vi "Start.vi"(8 "error in (no error)":errorcluster, 10 "Message in":refnum<class "StartMessage.lvclass">, 11 "Galvo in":refnum<class "ImagingModeSPIM.lvclass">) -> (0 "error out":errorcluster, 3 "Galvo out":refnum<class "ImagingModeSPIM.lvclass">)   [LabVIEW 2012, in "ImagingModeSPIM.lvclass"]
doc: "This member function is called when the statemachine in the run.vi receives an 'start' command. It relays the message to all observers of the component.\n\nOverride this member function in your derived class if you need additional start functionality (but don't forget to call the parent method)."
uses:
  ImagingModeSPIM.lvclass
  <vilib>/Distrio/Murmex/StartMessage/StartMessage.lvclass
  <vilib>/Distrio/Murmex/Murmex/Murmex.lvclass
  <vilib>/Distrio/Murmex/StartMessage/run mode enum.ctl
  <vilib>/Distrio/Murmex/ProceedMessage/ProceedMessage.lvclass
  ImagingModeSPIM.lvclass/ImagingModeSPIM.ctl
  <vilib>/Distrio/Murmex/StartMessage/Get run mode.vi
panel:
  # "This member function is called when the statemachine in the run.vi receives an 'start' command. It relays the message to all observers of the component.\n\nOverride this member function in your derived class if you need additional start functionality (but don't forget to call the parent method)."
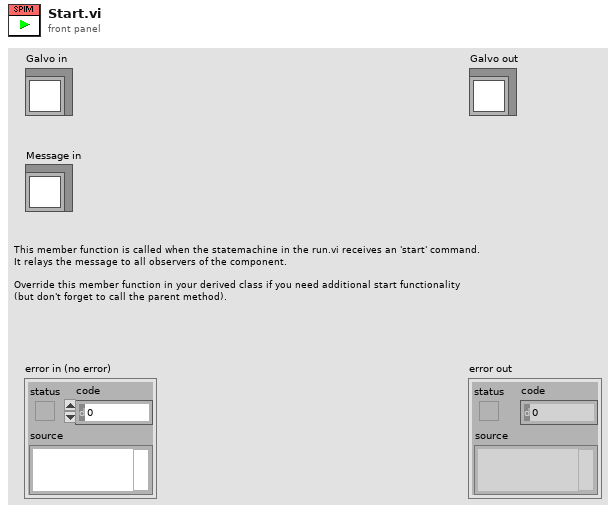
[diagram p1: front panel]
types:
  T1 = typedef "Murmex.lvlib/StartMessage.lvclass/run mode enum.ctl" = enum16{"infinite", "finite"}
  T2 = enum8{"Enabled", "Disabled", "Disabled and Grayed Out"}
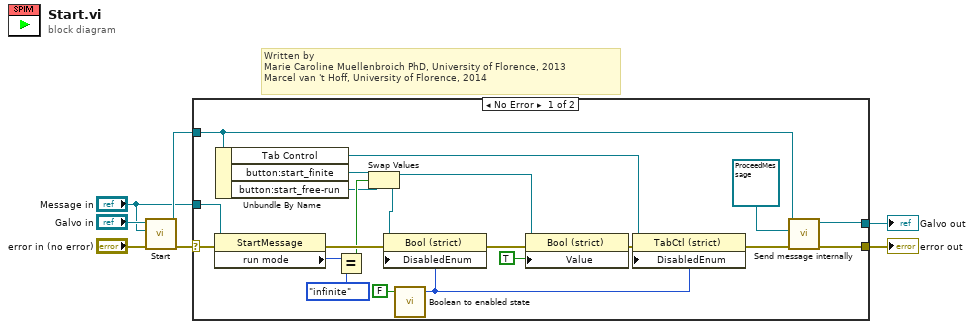
[diagram p0: block diagram]
diagram:
  # "Written by \nMarie Caroline Muellenbroich PhD, University of Florence, 2013 \nMarcel van 't Hoff, University of Florence, 2014"
  n1 = call-parent "Start.vi"("error in (no error)"="error in (no error)", "Message in"="Message in", "Murmex in"="Galvo in") -> ("error out"=w4:errorcluster, "Murmex out"=w5:refnum<class "ImagingModeSPIM.lvclass">)  [unwired: 7 in]
  n2 = case shown="No Error" w4 {
    selector: w4 -> [w25 w30]
    tunnel: w5 -> [w24 w29]
    tunnel: [w28 w30] -> w3
    tunnel: [w27 w29] -> w2
    tunnel: "Message in" -> [w26 _]
    frame No Error {
      n3 = property class="StartMessage"(reference=w26, error in=w25) -> (error out=w20:errorcluster, "run mode"=w23:T1)  [unwired: 1 out]
      n4 = Unbundle By Name(w24) -> ("Tab Control"=w19:refnum<vi>, "button:start_finite"=w15:refnum<vi>, "button:start_free-run"=w14:refnum<vi>)
      n5 = Equal?(x=w23, y=run_mode_enum."infinite" ("run mode")) -> (x = y?=w16:bool)
      n6 = Swap Values(12:w15, 13:w16, 14:w14) -> (1:w10:refnum<vi>, 3:w9:refnum<vi>)
      n7 = call <vilib>:"Boolean to enabled state.vi"("boolean in"=FALSE) -> ("enabled status out"=w18:T2)  [unwired: 4 in]
      n8 = property class="Bool (strict)"(reference=w9, error in=w20, "DisabledEnum"=w18) -> (error out=w12:errorcluster)  [unwired: 1 out]
      n9 = property class="Bool (strict)"(reference=w10, error in=w12, "Value"=TRUE) -> (error out=w11:errorcluster)  [unwired: 1 out]
      n10 = property class="TabCtl (strict)"(reference=w19, error in=w11, "DisabledEnum"=w18) -> (error out=w17:errorcluster)  [unwired: 1 out]
      n11 = call <vilib>:"Send message internally.vi"("error in (no error)"=w17, "Message"=refnum<class "ProceedMessage.lvclass"> refnum ("Murmex.lvlib:ProceedMessage"), "Murmex in"=w24) -> ("error out"=w28:errorcluster, "Murmex out"=w27:refnum<class "ImagingModeSPIM.lvclass">)  [unwired: 7 in]
    }
    frame Error {
    }
  }
  "error out" <- w3
  "Galvo out" <- w2
